vi "ClientTCPIP.vi"(9 "timeout \nms (60000)":i32, 10 "port":u16, 11 "Input String":string) -> (2 "error out":errorcluster, 3 "Output Data":string)   [LabVIEW 2023]
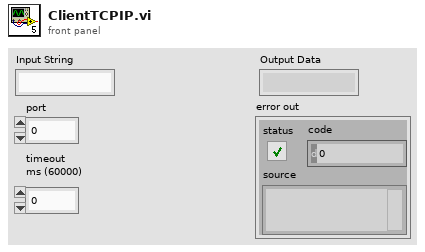
[diagram p1: front panel]
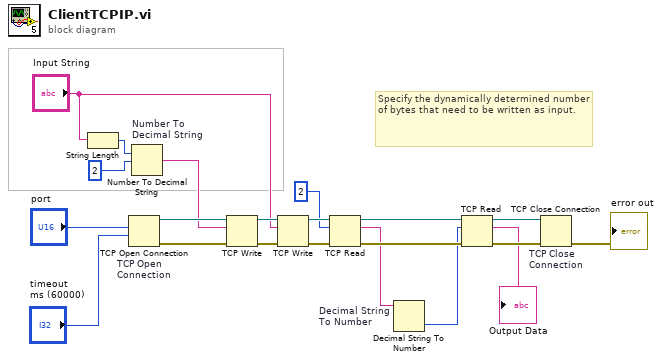
[diagram p0: block diagram]
diagram:
  # "Specify the dynamically determined number of bytes that need to be written as input."
  n1 = String Length(string="Input String") -> (length=w7:i32)
  n2 = TCP Open Connection "TCP Open\nConnection"(remote port or service name="port", timeout ms (60000)="timeout \nms (60000)") -> (connection ID=w20:refnum<k5>, error out=w21:errorcluster)  [unwired: 3 in]
  n3 = Number To Decimal String "Number To \nDecimal String"(number=w7, width (-)=i16 2) -> (decimal integer string=w5:string)
  n4 = TCP Write(connection ID=w20, data in=w5, error in (no error)=w21) -> (connection ID out=w14:refnum<k5>, error out=w19:errorcluster)  [unwired: 1 in, 1 out]
  n5 = TCP Write(connection ID=w14, data in="Input String", error in (no error)=w19) -> (connection ID out=w13:refnum<k5>, error out=w12:errorcluster)  [unwired: 1 in, 1 out]
  n6 = TCP Read(connection ID=w13, bytes to read=2, error in (no error)=w12) -> (connection ID out=w17:refnum<k5>, data out=w10:string, error out=w18:errorcluster)  [unwired: 2 in]
  n7 = Decimal String To Number "Decimal String\nTo Number"(string=w10) -> (number=w9:i32)  [unwired: 2 in, 1 out]
  n8 = TCP Read(connection ID=w17, bytes to read=w9, error in (no error)=w18) -> (connection ID out=w15:refnum<k5>, data out=→"Output Data":string, error out=w16:errorcluster)  [unwired: 2 in]
  n9 = TCP Close Connection "TCP Close \nConnection"(connection ID=w15, error in (no error)=w16) -> (error out=→"error out":errorcluster)  [unwired: 1 in, 1 out]
